vi "Deserialize Serial IO Class.vi"(7 "Formatter":refnum<class "Formatter.lvclass">, 8 "error in":errorcluster, 10 "cfg path":path, 11 "Serial IO in":refnum<class "Serial IO.lvclass">) -> (0 "error out":errorcluster, 1 "text":string, 3 "Serial IO out":refnum<class "Serial IO.lvclass">)   [LabVIEW 2012]
doc: "Deserialize Serial IO class from file."
uses:
  <userlib>/Serialization/JSON Deserializer/JSON Deserializer.lvclass
  <userlib>/Serialization/Deserializer/Deserializer.lvclass
  Serial IO.lvclass
  <userlib>/Serialization/Formatter/Formatter.lvclass
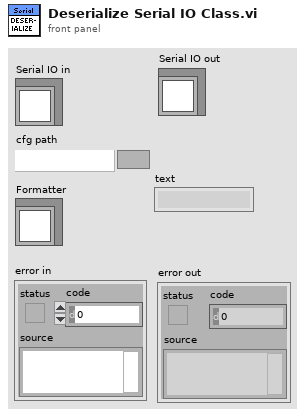
[diagram p1: front panel]
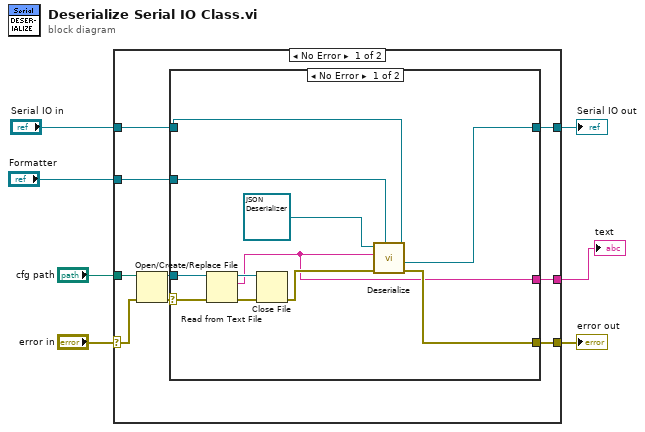
[diagram p0: block diagram]
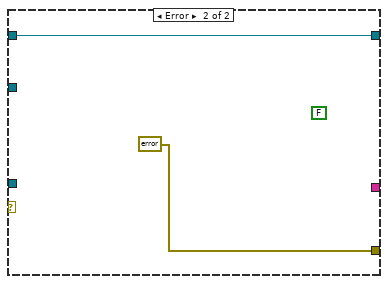
[diagram p2: hidden frame]
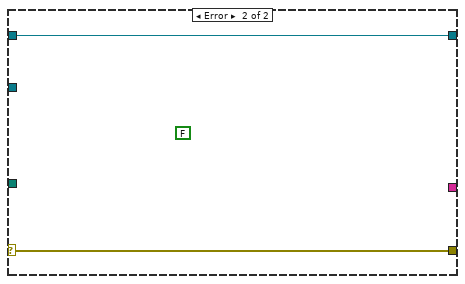
[diagram p3: hidden frame]
diagram:
  n1 = case shown="No Error" "error in" {
    selector: "error in" -> [w15 w31]
    tunnel: [w10 w31] -> w6
    tunnel: [w11 w30] -> w4
    tunnel: "Serial IO in" -> [w12 w30]
    tunnel: "cfg path" -> [w16 _]
    tunnel: "Formatter" -> [w9 _]
    tunnel: [w8 _] -> w1
    frame No Error {
      n2 = Open/Create/Replace File(file path (use dialog)=w16, error in=w15) -> (refnum out=w13:refnum<file>, error out=w14:errorcluster)  [unwired: 4 in, 1 out]
      n3 = case shown="No Error" w14 {
        selector: w14 -> [w27 _]
        tunnel: w13 -> [w26 _]
        tunnel: w12 -> [w24 w29]
        tunnel: [w23 w29] -> w11
        tunnel: [w19 errorcluster {"status"=FALSE, "code"=0, "source"=""} ("error out")] -> w10
        tunnel: w9 -> [w18 _]
        tunnel: [w17 _] -> w8
        frame No Error {
          n4 = Read from Text File(file (use dialog)=w26, error in=w27) -> (refnum out=w21:refnum<file>, text=w17:string, error out=w22:errorcluster)  [unwired: 2 in, 1 out]
          n5 = Close File(refnum=w21, error in=w22) -> (error out=w20:errorcluster)  [unwired: 1 out]
          n6 = call <userlib>:"Deserialize.vi"("Target Type (Serializable.lvclass)"=w24, "Formatter (defaults)"=w18, "error in (no error)"=w20, "String"=w17, "Deserializer"=refnum<class "JSON Deserializer.lvclass"> refnum ("JSON Deserializer.lvclass")) -> ("error out"=w19:errorcluster, "Serializable"=w23:refnum<class "Serializable.lvclass">)  [unwired: 4 in, 1 out]
        }
        frame Error {
          (unwired) FALSE
        }
      }
    }
    frame Error {
      (unwired) FALSE
    }
  }
  "error out" <- w6
  "Serial IO out" <- w4
  "text" <- w1
